vi "测试.vi"() -> ()   [LabVIEW 2016, in "中水三立SQL数据传输.lvlib"]
uses:
  access/access.lvclass
panel:
  in  "condition":string
  in  "columns":string[](array[string])=["ID", "MN", "CurTime", "PH", "ZD", "RJY", "DDL", "KMnO4", "NH4", "TP", "SW", "BZ"]
  in  "table":string="dbo.LS_Data"
  in  "停止":bool
  out "error out":errorcluster caption="错误输出"
  in  "error in (no error)":errorcluster caption="错误输入（无错误）"
  out "data":string[][](array[string])
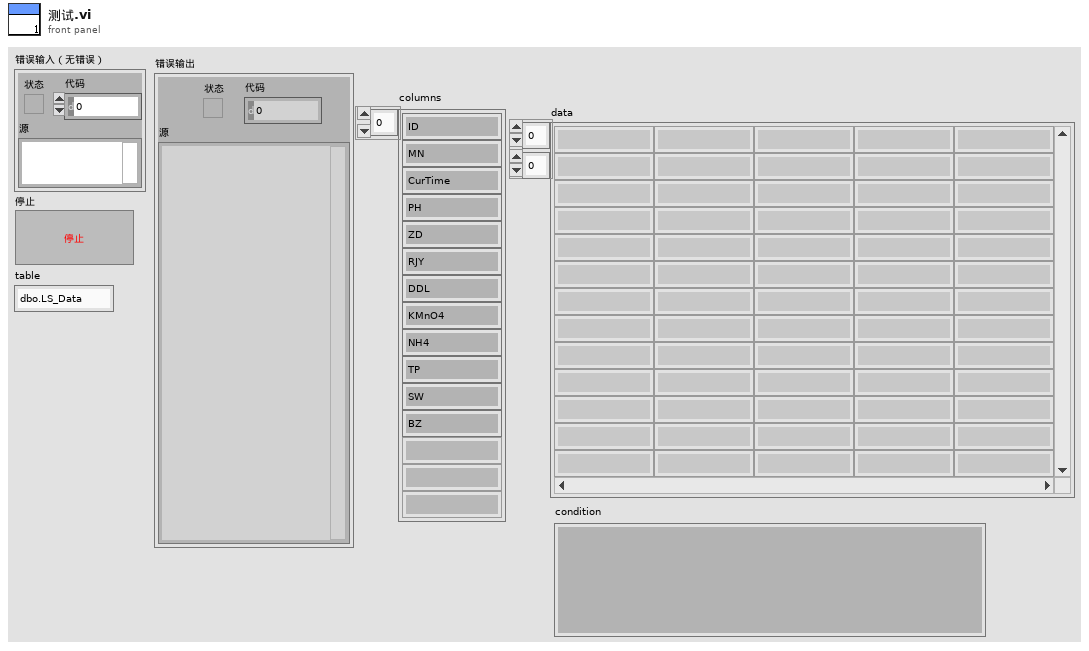
[diagram p1: front panel]
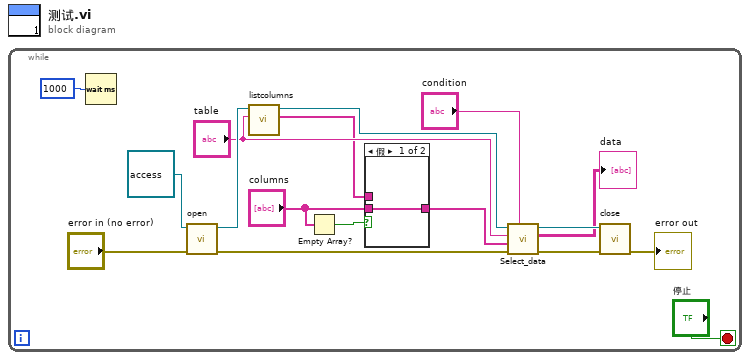
[diagram p0: block diagram]
diagram:
  n1 = while {
    stop <- "停止" stop-if-true
    n2 = Wait (ms)(milliseconds to wait=u32 1000 ("等待时间（毫秒）")) -> ()  [unwired: 1 out]
    n3 = call-dynamic "open.vi"("error in (no error)"="error in (no error)", "access 输入"=refnum<class "access.lvclass"> refnum ("中水三立SQL数据传输.lvlib:access.lvclass")) -> ("error out"=w15:errorcluster, "access 输出"=w8:refnum<class "access.lvclass">)  [unwired: 8 in]
    n4 = call-dynamic "listcolumns.vi"("table"="table", "access 输入"=w8) -> ("columns"=w3:string[], "access 输出"=w6:refnum<class "access.lvclass">)  [unwired: 7 in, 1 out]
    n5 = Empty Array?(array="columns") -> (empty?=w5:bool)
    n6 = case shown="假" w5 {
      tunnel: w3 -> [_ w19]
      tunnel: [w18 w19] -> w2
      tunnel: "columns" -> [w18 _]
      frame False {
      }
      frame True {
      }
    }
    n7 = call-dynamic "Select_data.vi"("condition"="condition", "error in (no error)"=w15, "columns"=w2, "table"="table", "access 输入"=w6) -> ("error out"=w14:errorcluster, "data"=→"data":string[][], "access 输出"=w16:refnum<class "access.lvclass">)  [unwired: 4 in]
    n8 = call-dynamic "close.vi"("error in (no error)"=w14, "access 输入"=w16) -> ("error out"=→"error out":errorcluster)  [unwired: 8 in, 1 out]
  }
